vi "ReadVI.vi"(0 "__args":cluster{"targetVi":string}) -> (1 "__return":string, 2 "__errStatus":bool, 3 "__errCode":i32, 4 "__errSource":string)   [LabVIEW 2014]
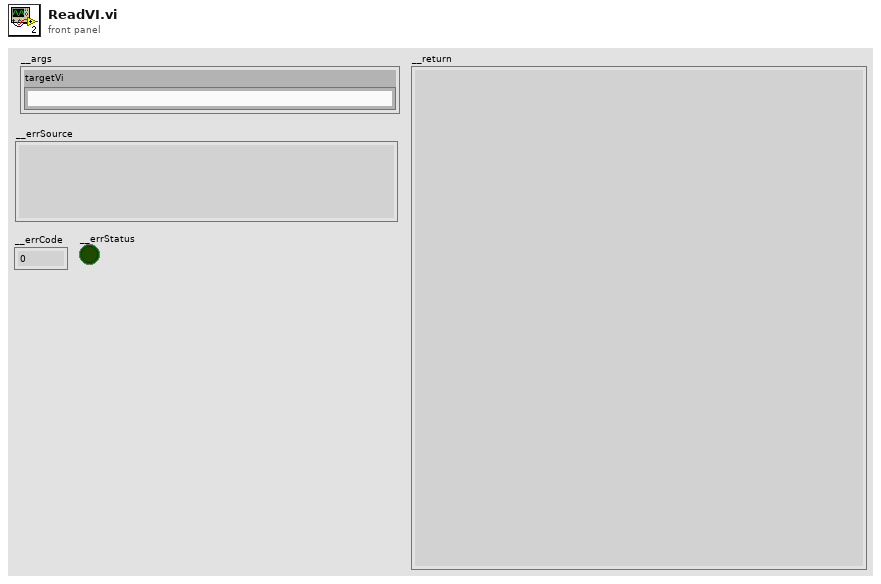
[diagram p1: front panel]
types:
  T1 = typedef "LVBoundsTypeDef.ctl" = cluster{"Width":u32, "Height":u32}
  T2 = typedef "LVPositionTypeDef.ctl" = cluster{"Left":i32, "Top":i32}
  T3 = typedef "LVRectTypeDef.ctl" = cluster{"Left":i16, "Top":i16, "Right":i16, "Bottom":i16}
  T4 = typedef "LVBreakpointStatusEnum.ctl" = enum8{"Cleared Break", "Enabled Break", "Disabled Break"}
  T5 = typedef "LVDataSocketStatusTypeDef.ctl" = cluster{"Code":enum32{"Invalid Status", "Unconnected", "Active", "Idle", "Error", "Connecting"}, "Text":string}
  T6 = typedef "LVKeyNavTypeDef.ctl" = cluster{"Control":bool, "Shift":bool, "Key":string}
  T7 = typedef "LVNumericRepresentation.ctl" = enum32{"Extended Precision", "Double Precision", "Single Precision", "Long", "Word", "Byte", "Unsigned Long", "Unsigned Word", "Unsigned Byte", "Complex Extended", "Complex Double", "Complex Single", "Quad", "Unsigned Quad", "Fixed-Point"}
  T8 = typedef "LVStringsAndValuesArrayTypeDef.ctl" = cluster{"String":string, "Value":ext}[]
  T9 = typedef "LVParallelSchedulesEnum.ctl" = enum8{"Dynamic decreasing", "Dynamic fixed size", "Static block", "Static block-cyclic"}
  T10 = typedef "LVMinMaxIncTypeDef.ctl" = cluster{"Minimum":dbl, "Maximum":dbl, "Increment":dbl}
  T11 = typedef "LVKeyTypeDef.ctl" = cluster{"Focus":bool, "Control":bool, "Shift":bool, "Key":string}
  T12 = typedef "LVOutOfRangeActionTypeDef.ctl" = cluster{"Out of Range Action Minimum":u8, "Out of Range Action Maximum":u8, "Out of Range Action Increment":u8}
  T13 = cluster{"Wire":cluster{"ClassID":u32, "ClassName":string, "IsOnBD?":bool, "Owner":cluster{bool, "UID":i32}, "OwningVI":refnum<vi>, "Bounds":T1, "Height":u32, "Width":u32, "Position":T2, "Left":i32, "Top":i32, "Selected":bool, "Bounds Rect":T3, "UID":i32, "BreakPtStatus":T4, "Desc":string, "Broken?":bool, "Joints[]":cluster{"Position":cluster{"h":i16, "v":i16}, "Flags":i32, "Type":enum32{"LooseEnd", "Endpoint", "Bend", "Junction"}, "Up Joint Index":i16, "Down Joint Index":i16, "Left Joint Index":i16, "Right Joint Index":i16}[], "Label":string, "Probe":refnum<vi>, "Terms[]":i32[], "Width":u32}[], cluster{"ClassID":u32, "ClassName":string, "IsOnBD?":bool, "Owner":cluster{bool, "UID":i32}, "OwningVI":refnum<vi>, "Bounds":T1, "Height":u32, "Width":u32, "Position":T2, "Left":i32, "Top":i32, "Selected":bool, "Bounds Rect":T3, "UID":i32, "Caption":string, "Coerce Dot?":bool, "Wire":i32, "Diagram":i32, "IsHidden":bool, "IsSource":bool, "Name":string}[], cluster{"ClassID":u32, "ClassName":string, "IsOnBD?":bool, "Owner":cluster{bool, "UID":i32}, "OwningVI":refnum<vi>, "Bounds":T1, "Height":u32, "Width":u32, "Position":T2, "Left":i32, "Top":i32, "Selected":bool, "Bounds Rect":T3, "UID":i32, "Input?":bool, "Name":string, "Term":i32}[], cluster{"ClassID":u32, "ClassName":string, "IsOnBD?":bool, "Owner":cluster{bool, "UID":i32}, "OwningVI":refnum<vi>, "Bounds":T1, "Height":u32, "Width":u32, "Position":T2, "Left":i32, "Top":i32, "Selected":bool, "Bounds Rect":T3, "UID":i32, "BreakPtStatus":T4, "Desc":string, "Label":string, "Style":string, "Terms[]":i32[], "FormExpr":string, "FormulaParameters[]":i32[]}[], cluster{"ClassID":u32, "ClassName":string, "IsOnBD?":bool, "Owner":cluster{bool, "UID":i32}, "OwningVI":refnum<vi>, "Bounds":T1, "Height":u32, "Width":u32, "Position":T2, "Left":i32, "Top":i32, "Selected":bool, "Bounds Rect":T3, "UID":i32, "BreakPtStatus":T4, "Desc":string, "Label":string, "Style":string, "Terms[]":i32[], "FormExpr":string, "FormulaParameters[]":i32[]}[], cluster{"ClassID":u32, "ClassName":string, "IsOnBD?":bool, "Owner":cluster{bool, "UID":i32}, "OwningVI":refnum<vi>, "Bounds":T1, "Height":u32, "Width":u32, "Position":T2, "Left":i32, "Top":i32, "Selected":bool, "Bounds Rect":T3, "UID":i32, "BreakPtStatus":T4, "Desc":string, "Label":string, "Style":string, "Terms[]":i32[], "TermHeight":i32, "Invert Inputs?[]":bool[], "Invert Output":bool, "Mode":u32}[], cluster{"ClassID":u32, "ClassName":string, "IsOnBD?":bool, "Owner":cluster{bool, "UID":i32}, "OwningVI":refnum<vi>, "Bounds":T1, "Height":u32, "Width":u32, "Position":T2, "Left":i32, "Top":i32, "Selected":bool, "Bounds Rect":T3, "UID":i32, "BreakPtStatus":T4, "Desc":string, "Label":string, "Style":string, "Terms[]":i32[], "TermHeight":i32, "InputCnt":i32, "InputTerms[]":i32[]}[], cluster{"ClassID":u32, "ClassName":string, "IsOnBD?":bool, "Owner":cluster{bool, "UID":i32}, "OwningVI":refnum<vi>, "Bounds":T1, "Height":u32, "Width":u32, "Position":T2, "Left":i32, "Top":i32, "Selected":bool, "Bounds Rect":T3, "UID":i32, "BreakPtStatus":T4, "Desc":string, "Label":string, "Style":string, "Terms[]":i32[], "TermHeight":i32, "OutputCnt":i32, "OutputTerms[]":i32[]}[], cluster{"ClassID":u32, "ClassName":string, "IsOnBD?":bool, "Owner":cluster{bool, "UID":i32}, "OwningVI":refnum<vi>, "Bounds":T1, "Height":u32, "Width":u32, "Position":T2, "Left":i32, "Top":i32, "Selected":bool, "Bounds Rect":T3, "UID":i32, "Auto-Update":bool, "Blinking":bool, "BuiltInMouseWheelSupport":enum16{"None", "On Hover", "On Key Focus", "On Hover or Key Focus"}, "Caption":refnum<vi>, "ControlIndex":i32, "CtrlRefNodes":refnum<vi>[], "FPB.BindingType":enum32{"Unbound", "Bound To PSP URL", "Bound To Variable Shortcut"}, "FPB.LEDVisible":bool, "FPB.Mode":enum32{"No PSP", "Read", "Write", "Write & Read"}, "FPB.URL":string, "FPB.Status":T5, "DtSktEnbld":bool, "DtSktTagVisible":bool, "DtSktMode":enum32{"No DataSocket", "Publish", "Subscribe", "Publish & Subscribe"}, "DtSktStatus":T5, "DtSktURL":string, "DefVal":variant, "Desc":string, "DisabledEnum":enum8{"Enabled", "Disabled", "Disabled and Grayed Out"}, "KeyNav":T6, "GrowInfo":cluster{"Can Grow Horiz":bool, "Can Grow Vert":bool, "Min Horiz":i16, "Min Vert":i16, "Max Horiz":i16, "Max Vert":i16}, "GrowInfoHorizOnly":bool, "GrowInfoVertOnly":bool, "GrowInfoMaxHoriz":i16, "GrowInfoMaxVert":i16, "GrowInfoMinHoriz":i16, "GrowInfoMinVert":i16, "HasCaption":bool, "Indicator":bool, "InvokeNodes":refnum<vi>[], "IsOnConPane":bool, "Typedef?":enum32{"not a typedef", "typedef", "strict typedef", "class private data"}, "Key Focus":bool, "Label":string, "Locals":refnum<vi>[], "OwningPane":refnum<vi>, "PropNodes":refnum<vi>[], "SkipTabbing":bool, "Style":u32, "SyncDisp":bool, "Terminal":i32, "TipStrip":string, "Typedef Path":path, "Typedef VI":refnum<vi>, "Value":variant, "Visible":bool, "Container Bounds":T1, "Height":u32, "Width":u32, "Is XControl?":bool, "Adapt To Source":bool, "Data Range":T10, "Increment":dbl, "Maximum":dbl, "Minimum":dbl, "DecKeyBind":T11, "IncKeyBind":T11, "Rep":T7, "OutOfRngAction":T12, "OutOfRngActInc":u8, "OutOfRngActMax":u8, "OutOfRngActMin":u8, "UnitLabel":refnum<vi>}[], cluster{"ClassID":u32, "ClassName":string, "IsOnBD?":bool, "Owner":cluster{bool, "UID":i32}, "OwningVI":refnum<vi>, "Bounds":T1, "Height":u32, "Width":u32, "Position":T2, "Left":i32, "Top":i32, "Selected":bool, "Bounds Rect":T3, "UID":i32, "Auto-Update":bool, "Blinking":bool, "BuiltInMouseWheelSupport":enum16{"None", "On Hover", "On Key Focus", "On Hover or Key Focus"}, "Caption":refnum<vi>, "ControlIndex":i32, "CtrlRefNodes":refnum<vi>[], "FPB.BindingType":enum32{"Unbound", "Bound To PSP URL", "Bound To Variable Shortcut"}, "FPB.LEDVisible":bool, "FPB.Mode":enum32{"No PSP", "Read", "Write", "Write & Read"}, "FPB.URL":string, "FPB.Status":T5, "DtSktEnbld":bool, "DtSktTagVisible":bool, "DtSktMode":enum32{"No DataSocket", "Publish", "Subscribe", "Publish & Subscribe"}, "DtSktStatus":T5, "DtSktURL":string, "DefVal":variant, "Desc":string, "DisabledEnum":enum8{"Enabled", "Disabled", "Disabled and Grayed Out"}, "KeyNav":T6, "GrowInfo":cluster{"Can Grow Horiz":bool, "Can Grow Vert":bool, "Min Horiz":i16, "Min Vert":i16, "Max Horiz":i16, "Max Vert":i16}, "GrowInfoHorizOnly":bool, "GrowInfoVertOnly":bool, "GrowInfoMaxHoriz":i16, "GrowInfoMaxVert":i16, "GrowInfoMinHoriz":i16, "GrowInfoMinVert":i16, "HasCaption":bool, "Indicator":bool, "InvokeNodes":refnum<vi>[], "IsOnConPane":bool, "Typedef?":enum32{"not a typedef", "typedef", "strict typedef", "class private data"}, "Key Focus":bool, "Label":string, "Locals":refnum<vi>[], "OwningPane":refnum<vi>, "PropNodes":refnum<vi>[], "SkipTabbing":bool, "Style":u32, "SyncDisp":bool, "Terminal":i32, "TipStrip":string, "Typedef Path":path, "Typedef VI":refnum<vi>, "Value":variant, "Visible":bool, "Container Bounds":T1, "Height":u32, "Width":u32, "Is XControl?":bool, "AllObjs[]":refnum<vi>[], "AutoSize":u32, "ClusterSize":T1, "ClustHeight":u32, "ClustWidth":u32, "Color":u32, "Controls[]":i32[], "Decos[]":refnum<vi>[]}[], cluster{"ClassID":u32, "ClassName":string, "IsOnBD?":bool, "Owner":cluster{bool, "UID":i32}, "OwningVI":refnum<vi>, "Bounds":T1, "Height":u32, "Width":u32, "Position":T2, "Left":i32, "Top":i32, "Selected":bool, "Bounds Rect":T3, "UID":i32, "Auto-Update":bool, "Blinking":bool, "BuiltInMouseWheelSupport":enum16{"None", "On Hover", "On Key Focus", "On Hover or Key Focus"}, "Caption":refnum<vi>, "ControlIndex":i32, "CtrlRefNodes":refnum<vi>[], "FPB.BindingType":enum32{"Unbound", "Bound To PSP URL", "Bound To Variable Shortcut"}, "FPB.LEDVisible":bool, "FPB.Mode":enum32{"No PSP", "Read", "Write", "Write & Read"}, "FPB.URL":string, "FPB.Status":T5, "DtSktEnbld":bool, "DtSktTagVisible":bool, "DtSktMode":enum32{"No DataSocket", "Publish", "Subscribe", "Publish & Subscribe"}, "DtSktStatus":T5, "DtSktURL":string, "DefVal":variant, "Desc":string, "DisabledEnum":enum8{"Enabled", "Disabled", "Disabled and Grayed Out"}, "KeyNav":T6, "GrowInfo":cluster{"Can Grow Horiz":bool, "Can Grow Vert":bool, "Min Horiz":i16, "Min Vert":i16, "Max Horiz":i16, "Max Vert":i16}, "GrowInfoHorizOnly":bool, "GrowInfoVertOnly":bool, "GrowInfoMaxHoriz":i16, "GrowInfoMaxVert":i16, "GrowInfoMinHoriz":i16, "GrowInfoMinVert":i16, "HasCaption":bool, "Indicator":bool, "InvokeNodes":refnum<vi>[], "IsOnConPane":bool, "Typedef?":enum32{"not a typedef", "typedef", "strict typedef", "class private data"}, "Key Focus":bool, "Label":string, "Locals":refnum<vi>[], "OwningPane":refnum<vi>, "PropNodes":refnum<vi>[], "SkipTabbing":bool, "Style":u32, "SyncDisp":bool, "Terminal":i32, "TipStrip":string, "Typedef Path":path, "Typedef VI":refnum<vi>, "Value":variant, "Visible":bool, "Container Bounds":T1, "Height":u32, "Width":u32, "Is XControl?":bool, "Array Element":refnum<vi>, "HorizScroll":bool, "Index Values":u32[], "Index Visible":bool, "Number of Columns":u32, "NumDims":u32, "Number of Rows":u32, "Selection Size []":u32[], "Selection Start []":u32[], "VertScroll":bool}[], cluster{"ClassID":u32, "ClassName":string, "IsOnBD?":bool, "Owner":cluster{bool, "UID":i32}, "OwningVI":refnum<vi>, "Bounds":T1, "Height":u32, "Width":u32, "Position":T2, "Left":i32, "Top":i32, "Selected":bool, "Bounds Rect":T3, "UID":i32, "Auto-Update":bool, "Desc":string, "Typedef?":enum32{"not a typedef", "typedef", "strict typedef", "class private data"}, "Label":string, "Terminal":i32, "TipStrip":string, "Typedef Path":path, "Typedef VI":refnum<vi>, "Value":variant, "Adapt To Entered Data":bool, "Representation":T7, "DigDisp":refnum<vi>, "Items[]":string[], "Allow Undefined Values?":bool, "Strings And Values[]":T8}[], cluster{"ClassID":u32, "ClassName":string, "IsOnBD?":bool, "Owner":cluster{bool, "UID":i32}, "OwningVI":refnum<vi>, "Bounds":T1, "Height":u32, "Width":u32, "Position":T2, "Left":i32, "Top":i32, "Selected":bool, "Bounds Rect":T3, "UID":i32, "BreakPtStatus":T4, "Desc":string, "Label":string, "Style":string, "Terms[]":i32[], "BadSubVILinkage":bool, "GrowTerms":string[], "SkipSbrtCall":bool, "CloseFPAfterCall":bool, "Open FP On Load":bool, "Show FP On Call":bool, "SuspendOnCall":bool, "TermVis":bool, "VIName":string, "VIPath":path, "VI Ref":refnum<vi>, "ViewAsIcon":bool}[], cluster{"ClassID":u32, "ClassName":string, "IsOnBD?":bool, "Owner":cluster{bool, "UID":i32}, "OwningVI":refnum<vi>, "Bounds":T1, "Height":u32, "Width":u32, "Position":T2, "Left":i32, "Top":i32, "Selected":bool, "Bounds Rect":T3, "UID":i32, "InsideTerms[]":i32[], "Outer Term":i32, "RightReg":i32}[], cluster{"ClassID":u32, "ClassName":string, "IsOnBD?":bool, "Owner":cluster{bool, "UID":i32}, "OwningVI":refnum<vi>, "Bounds":T1, "Height":u32, "Width":u32, "Position":T2, "Left":i32, "Top":i32, "Selected":bool, "Bounds Rect":T3, "UID":i32, "InsideTerms[]":i32[], "Outer Term":i32, "LeftRegs[]":i32[]}[], cluster{"ClassID":u32, "ClassName":string, "IsOnBD?":bool, "Owner":cluster{bool, "UID":i32}, "OwningVI":refnum<vi>, "Bounds":T1, "Height":u32, "Width":u32, "Position":T2, "Left":i32, "Top":i32, "Selected":bool, "Bounds Rect":T3, "UID":i32, "BreakPtStatus":T4, "Desc":string, "Label":string, "Style":string, "Terms[]":i32[], "AutoSize":bool, "Content Rect":T3, "Diagrams":refnum<vi>[], "Fix Contents":bool, "Frame Size":T1, "AutoSharedCloneAllocStrategyEnabled":bool, "PreAllocSharedClones":bool, "SubDiagLbl Vis":bool, "Tunnels[]":i32[], "Diagram":i32, "LpCounter":refnum<vi>, "ShiftRegs[]":i32[], "LpEndRef":refnum<vi>, "StopIfTrue":bool}[], cluster{"ClassID":u32, "ClassName":string, "IsOnBD?":bool, "Owner":cluster{bool, "UID":i32}, "OwningVI":refnum<vi>, "Bounds":T1, "Height":u32, "Width":u32, "Position":T2, "Left":i32, "Top":i32, "Selected":bool, "Bounds Rect":T3, "UID":i32, "BreakPtStatus":T4, "Desc":string, "Label":string, "Style":string, "Terms[]":i32[], "AutoSize":bool, "Content Rect":T3, "Diagrams":refnum<vi>[], "Fix Contents":bool, "Frame Size":T1, "AutoSharedCloneAllocStrategyEnabled":bool, "PreAllocSharedClones":bool, "SubDiagLbl Vis":bool, "Tunnels[]":i32[], "Diagram":i32, "LpCounter":refnum<vi>, "ShiftRegs[]":i32[], "ChunkSizeTunnel":refnum<vi>, "PTunnel":refnum<vi>, "HasConditionalTerm":bool, "DebuggingAllowed":bool, "IsParallelismEnabled":bool, "LpCount":refnum<vi>, "LpEndRef":refnum<vi>, "NumStaticParWorkers":i32, "ParallelSchedule":T9, "StopIfTrue":bool}[], cluster{"ClassID":u32, "ClassName":string, "IsOnBD?":bool, "Owner":cluster{bool, "UID":i32}, "OwningVI":refnum<vi>, "Bounds":T1, "Height":u32, "Width":u32, "Position":T2, "Left":i32, "Top":i32, "Selected":bool, "Bounds Rect":T3, "UID":i32, "AllObjs[]":refnum<vi>[], "BreakPtStatus":T4, "Color":u32, "Decos[]":refnum<vi>[], "FiringOrder":refnum<vi>[], "Nodes[]":refnum<vi>[], "SubDiag Label":refnum<vi>, "SubVIs[]":refnum<vi>[], "Wires[]":refnum<vi>[], "VisBounds":T1}[], cluster{"ClassID":u32, "ClassName":string, "IsOnBD?":bool, "Owner":cluster{bool, "UID":i32}, "OwningVI":refnum<vi>, "Bounds":T1, "Height":u32, "Width":u32, "Position":T2, "Left":i32, "Top":i32, "Selected":bool, "Bounds Rect":T3, "UID":i32, "AllObjs[]":refnum<vi>[], "Controls[]":i32[], "Decos[]":refnum<vi>[], "DeferPanUpdts":bool, "Panes[]":refnum<vi>[], "SelList[]":refnum<vi>[], "Splitters[]":refnum<vi>[]}[], cluster{"ClassID":u32, "ClassName":string, "IsOnBD?":bool, "Owner":cluster{bool, "UID":i32}, "OwningVI":refnum<vi>, "Bounds":T1, "Height":u32, "Width":u32, "Position":T2, "Left":i32, "Top":i32, "Selected":bool, "Bounds Rect":T3, "UID":i32, "InsideTerms[]":i32[], "Outer Term":i32}[]}
  T14 = cluster{"ClassID":u32, "ClassName":string, "IsOnBD?":bool, "Owner":cluster{bool, "UID":i32}, "OwningVI":refnum<vi>, "Bounds":T1, "Height":u32, "Width":u32, "Position":T2, "Left":i32, "Top":i32, "Selected":bool, "Bounds Rect":T3, "UID":i32, "BreakPtStatus":T4, "Desc":string, "Broken?":bool, "Joints[]":cluster{"Position":cluster{"h":i16, "v":i16}, "Flags":i32, "Type":enum32{"LooseEnd", "Endpoint", "Bend", "Junction"}, "Up Joint Index":i16, "Down Joint Index":i16, "Left Joint Index":i16, "Right Joint Index":i16}[], "Label":string, "Probe":refnum<vi>, "Terms[]":i32[], "Width":u32}[]
  T15 = cluster{"ClassID":u32, "ClassName":string, "IsOnBD?":bool, "Owner":cluster{bool, "UID":i32}, "OwningVI":refnum<vi>, "Bounds":T1, "Height":u32, "Width":u32, "Position":T2, "Left":i32, "Top":i32, "Selected":bool, "Bounds Rect":T3, "UID":i32, "Caption":string, "Coerce Dot?":bool, "Wire":i32, "Diagram":i32, "IsHidden":bool, "IsSource":bool, "Name":string}[]
  T16 = cluster{"ClassID":u32, "ClassName":string, "IsOnBD?":bool, "Owner":cluster{bool, "UID":i32}, "OwningVI":refnum<vi>, "Bounds":T1, "Height":u32, "Width":u32, "Position":T2, "Left":i32, "Top":i32, "Selected":bool, "Bounds Rect":T3, "UID":i32, "Input?":bool, "Name":string, "Term":i32}[]
  T17 = cluster{"ClassID":u32, "ClassName":string, "IsOnBD?":bool, "Owner":cluster{bool, "UID":i32}, "OwningVI":refnum<vi>, "Bounds":T1, "Height":u32, "Width":u32, "Position":T2, "Left":i32, "Top":i32, "Selected":bool, "Bounds Rect":T3, "UID":i32, "BreakPtStatus":T4, "Desc":string, "Label":string, "Style":string, "Terms[]":i32[], "FormExpr":string, "FormulaParameters[]":i32[]}[]
  T18 = cluster{"ClassID":u32, "ClassName":string, "IsOnBD?":bool, "Owner":cluster{bool, "UID":i32}, "OwningVI":refnum<vi>, "Bounds":T1, "Height":u32, "Width":u32, "Position":T2, "Left":i32, "Top":i32, "Selected":bool, "Bounds Rect":T3, "UID":i32, "BreakPtStatus":T4, "Desc":string, "Label":string, "Style":string, "Terms[]":i32[], "TermHeight":i32, "Invert Inputs?[]":bool[], "Invert Output":bool, "Mode":u32}[]
  T19 = cluster{"ClassID":u32, "ClassName":string, "IsOnBD?":bool, "Owner":cluster{bool, "UID":i32}, "OwningVI":refnum<vi>, "Bounds":T1, "Height":u32, "Width":u32, "Position":T2, "Left":i32, "Top":i32, "Selected":bool, "Bounds Rect":T3, "UID":i32, "BreakPtStatus":T4, "Desc":string, "Label":string, "Style":string, "Terms[]":i32[], "TermHeight":i32, "InputCnt":i32, "InputTerms[]":i32[]}[]
  T20 = cluster{"ClassID":u32, "ClassName":string, "IsOnBD?":bool, "Owner":cluster{bool, "UID":i32}, "OwningVI":refnum<vi>, "Bounds":T1, "Height":u32, "Width":u32, "Position":T2, "Left":i32, "Top":i32, "Selected":bool, "Bounds Rect":T3, "UID":i32, "BreakPtStatus":T4, "Desc":string, "Label":string, "Style":string, "Terms[]":i32[], "TermHeight":i32, "OutputCnt":i32, "OutputTerms[]":i32[]}[]
  T21 = cluster{"ClassID":u32, "ClassName":string, "IsOnBD?":bool, "Owner":cluster{bool, "UID":i32}, "OwningVI":refnum<vi>, "Bounds":T1, "Height":u32, "Width":u32, "Position":T2, "Left":i32, "Top":i32, "Selected":bool, "Bounds Rect":T3, "UID":i32, "Auto-Update":bool, "Blinking":bool, "BuiltInMouseWheelSupport":enum16{"None", "On Hover", "On Key Focus", "On Hover or Key Focus"}, "Caption":refnum<vi>, "ControlIndex":i32, "CtrlRefNodes":refnum<vi>[], "FPB.BindingType":enum32{"Unbound", "Bound To PSP URL", "Bound To Variable Shortcut"}, "FPB.LEDVisible":bool, "FPB.Mode":enum32{"No PSP", "Read", "Write", "Write & Read"}, "FPB.URL":string, "FPB.Status":T5, "DtSktEnbld":bool, "DtSktTagVisible":bool, "DtSktMode":enum32{"No DataSocket", "Publish", "Subscribe", "Publish & Subscribe"}, "DtSktStatus":T5, "DtSktURL":string, "DefVal":variant, "Desc":string, "DisabledEnum":enum8{"Enabled", "Disabled", "Disabled and Grayed Out"}, "KeyNav":T6, "GrowInfo":cluster{"Can Grow Horiz":bool, "Can Grow Vert":bool, "Min Horiz":i16, "Min Vert":i16, "Max Horiz":i16, "Max Vert":i16}, "GrowInfoHorizOnly":bool, "GrowInfoVertOnly":bool, "GrowInfoMaxHoriz":i16, "GrowInfoMaxVert":i16, "GrowInfoMinHoriz":i16, "GrowInfoMinVert":i16, "HasCaption":bool, "Indicator":bool, "InvokeNodes":refnum<vi>[], "IsOnConPane":bool, "Typedef?":enum32{"not a typedef", "typedef", "strict typedef", "class private data"}, "Key Focus":bool, "Label":string, "Locals":refnum<vi>[], "OwningPane":refnum<vi>, "PropNodes":refnum<vi>[], "SkipTabbing":bool, "Style":u32, "SyncDisp":bool, "Terminal":i32, "TipStrip":string, "Typedef Path":path, "Typedef VI":refnum<vi>, "Value":variant, "Visible":bool, "Container Bounds":T1, "Height":u32, "Width":u32, "Is XControl?":bool, "Adapt To Source":bool, "Data Range":T10, "Increment":dbl, "Maximum":dbl, "Minimum":dbl, "DecKeyBind":T11, "IncKeyBind":T11, "Rep":T7, "OutOfRngAction":T12, "OutOfRngActInc":u8, "OutOfRngActMax":u8, "OutOfRngActMin":u8, "UnitLabel":refnum<vi>}[]
  T22 = cluster{"ClassID":u32, "ClassName":string, "IsOnBD?":bool, "Owner":cluster{bool, "UID":i32}, "OwningVI":refnum<vi>, "Bounds":T1, "Height":u32, "Width":u32, "Position":T2, "Left":i32, "Top":i32, "Selected":bool, "Bounds Rect":T3, "UID":i32, "Auto-Update":bool, "Blinking":bool, "BuiltInMouseWheelSupport":enum16{"None", "On Hover", "On Key Focus", "On Hover or Key Focus"}, "Caption":refnum<vi>, "ControlIndex":i32, "CtrlRefNodes":refnum<vi>[], "FPB.BindingType":enum32{"Unbound", "Bound To PSP URL", "Bound To Variable Shortcut"}, "FPB.LEDVisible":bool, "FPB.Mode":enum32{"No PSP", "Read", "Write", "Write & Read"}, "FPB.URL":string, "FPB.Status":T5, "DtSktEnbld":bool, "DtSktTagVisible":bool, "DtSktMode":enum32{"No DataSocket", "Publish", "Subscribe", "Publish & Subscribe"}, "DtSktStatus":T5, "DtSktURL":string, "DefVal":variant, "Desc":string, "DisabledEnum":enum8{"Enabled", "Disabled", "Disabled and Grayed Out"}, "KeyNav":T6, "GrowInfo":cluster{"Can Grow Horiz":bool, "Can Grow Vert":bool, "Min Horiz":i16, "Min Vert":i16, "Max Horiz":i16, "Max Vert":i16}, "GrowInfoHorizOnly":bool, "GrowInfoVertOnly":bool, "GrowInfoMaxHoriz":i16, "GrowInfoMaxVert":i16, "GrowInfoMinHoriz":i16, "GrowInfoMinVert":i16, "HasCaption":bool, "Indicator":bool, "InvokeNodes":refnum<vi>[], "IsOnConPane":bool, "Typedef?":enum32{"not a typedef", "typedef", "strict typedef", "class private data"}, "Key Focus":bool, "Label":string, "Locals":refnum<vi>[], "OwningPane":refnum<vi>, "PropNodes":refnum<vi>[], "SkipTabbing":bool, "Style":u32, "SyncDisp":bool, "Terminal":i32, "TipStrip":string, "Typedef Path":path, "Typedef VI":refnum<vi>, "Value":variant, "Visible":bool, "Container Bounds":T1, "Height":u32, "Width":u32, "Is XControl?":bool, "AllObjs[]":refnum<vi>[], "AutoSize":u32, "ClusterSize":T1, "ClustHeight":u32, "ClustWidth":u32, "Color":u32, "Controls[]":i32[], "Decos[]":refnum<vi>[]}[]
  T23 = cluster{"ClassID":u32, "ClassName":string, "IsOnBD?":bool, "Owner":cluster{bool, "UID":i32}, "OwningVI":refnum<vi>, "Bounds":T1, "Height":u32, "Width":u32, "Position":T2, "Left":i32, "Top":i32, "Selected":bool, "Bounds Rect":T3, "UID":i32, "Auto-Update":bool, "Blinking":bool, "BuiltInMouseWheelSupport":enum16{"None", "On Hover", "On Key Focus", "On Hover or Key Focus"}, "Caption":refnum<vi>, "ControlIndex":i32, "CtrlRefNodes":refnum<vi>[], "FPB.BindingType":enum32{"Unbound", "Bound To PSP URL", "Bound To Variable Shortcut"}, "FPB.LEDVisible":bool, "FPB.Mode":enum32{"No PSP", "Read", "Write", "Write & Read"}, "FPB.URL":string, "FPB.Status":T5, "DtSktEnbld":bool, "DtSktTagVisible":bool, "DtSktMode":enum32{"No DataSocket", "Publish", "Subscribe", "Publish & Subscribe"}, "DtSktStatus":T5, "DtSktURL":string, "DefVal":variant, "Desc":string, "DisabledEnum":enum8{"Enabled", "Disabled", "Disabled and Grayed Out"}, "KeyNav":T6, "GrowInfo":cluster{"Can Grow Horiz":bool, "Can Grow Vert":bool, "Min Horiz":i16, "Min Vert":i16, "Max Horiz":i16, "Max Vert":i16}, "GrowInfoHorizOnly":bool, "GrowInfoVertOnly":bool, "GrowInfoMaxHoriz":i16, "GrowInfoMaxVert":i16, "GrowInfoMinHoriz":i16, "GrowInfoMinVert":i16, "HasCaption":bool, "Indicator":bool, "InvokeNodes":refnum<vi>[], "IsOnConPane":bool, "Typedef?":enum32{"not a typedef", "typedef", "strict typedef", "class private data"}, "Key Focus":bool, "Label":string, "Locals":refnum<vi>[], "OwningPane":refnum<vi>, "PropNodes":refnum<vi>[], "SkipTabbing":bool, "Style":u32, "SyncDisp":bool, "Terminal":i32, "TipStrip":string, "Typedef Path":path, "Typedef VI":refnum<vi>, "Value":variant, "Visible":bool, "Container Bounds":T1, "Height":u32, "Width":u32, "Is XControl?":bool, "Array Element":refnum<vi>, "HorizScroll":bool, "Index Values":u32[], "Index Visible":bool, "Number of Columns":u32, "NumDims":u32, "Number of Rows":u32, "Selection Size []":u32[], "Selection Start []":u32[], "VertScroll":bool}[]
  T24 = cluster{"ClassID":u32, "ClassName":string, "IsOnBD?":bool, "Owner":cluster{bool, "UID":i32}, "OwningVI":refnum<vi>, "Bounds":T1, "Height":u32, "Width":u32, "Position":T2, "Left":i32, "Top":i32, "Selected":bool, "Bounds Rect":T3, "UID":i32, "Auto-Update":bool, "Desc":string, "Typedef?":enum32{"not a typedef", "typedef", "strict typedef", "class private data"}, "Label":string, "Terminal":i32, "TipStrip":string, "Typedef Path":path, "Typedef VI":refnum<vi>, "Value":variant, "Adapt To Entered Data":bool, "Representation":T7, "DigDisp":refnum<vi>, "Items[]":string[], "Allow Undefined Values?":bool, "Strings And Values[]":T8}[]
  T25 = cluster{"ClassID":u32, "ClassName":string, "IsOnBD?":bool, "Owner":cluster{bool, "UID":i32}, "OwningVI":refnum<vi>, "Bounds":T1, "Height":u32, "Width":u32, "Position":T2, "Left":i32, "Top":i32, "Selected":bool, "Bounds Rect":T3, "UID":i32, "BreakPtStatus":T4, "Desc":string, "Label":string, "Style":string, "Terms[]":i32[], "BadSubVILinkage":bool, "GrowTerms":string[], "SkipSbrtCall":bool, "CloseFPAfterCall":bool, "Open FP On Load":bool, "Show FP On Call":bool, "SuspendOnCall":bool, "TermVis":bool, "VIName":string, "VIPath":path, "VI Ref":refnum<vi>, "ViewAsIcon":bool}[]
  T26 = cluster{"ClassID":u32, "ClassName":string, "IsOnBD?":bool, "Owner":cluster{bool, "UID":i32}, "OwningVI":refnum<vi>, "Bounds":T1, "Height":u32, "Width":u32, "Position":T2, "Left":i32, "Top":i32, "Selected":bool, "Bounds Rect":T3, "UID":i32, "InsideTerms[]":i32[], "Outer Term":i32, "RightReg":i32}[]
  T27 = cluster{"ClassID":u32, "ClassName":string, "IsOnBD?":bool, "Owner":cluster{bool, "UID":i32}, "OwningVI":refnum<vi>, "Bounds":T1, "Height":u32, "Width":u32, "Position":T2, "Left":i32, "Top":i32, "Selected":bool, "Bounds Rect":T3, "UID":i32, "InsideTerms[]":i32[], "Outer Term":i32, "LeftRegs[]":i32[]}[]
  T28 = cluster{"ClassID":u32, "ClassName":string, "IsOnBD?":bool, "Owner":cluster{bool, "UID":i32}, "OwningVI":refnum<vi>, "Bounds":T1, "Height":u32, "Width":u32, "Position":T2, "Left":i32, "Top":i32, "Selected":bool, "Bounds Rect":T3, "UID":i32, "BreakPtStatus":T4, "Desc":string, "Label":string, "Style":string, "Terms[]":i32[], "AutoSize":bool, "Content Rect":T3, "Diagrams":refnum<vi>[], "Fix Contents":bool, "Frame Size":T1, "AutoSharedCloneAllocStrategyEnabled":bool, "PreAllocSharedClones":bool, "SubDiagLbl Vis":bool, "Tunnels[]":i32[], "Diagram":i32, "LpCounter":refnum<vi>, "ShiftRegs[]":i32[], "LpEndRef":refnum<vi>, "StopIfTrue":bool}[]
  T29 = cluster{"ClassID":u32, "ClassName":string, "IsOnBD?":bool, "Owner":cluster{bool, "UID":i32}, "OwningVI":refnum<vi>, "Bounds":T1, "Height":u32, "Width":u32, "Position":T2, "Left":i32, "Top":i32, "Selected":bool, "Bounds Rect":T3, "UID":i32, "BreakPtStatus":T4, "Desc":string, "Label":string, "Style":string, "Terms[]":i32[], "AutoSize":bool, "Content Rect":T3, "Diagrams":refnum<vi>[], "Fix Contents":bool, "Frame Size":T1, "AutoSharedCloneAllocStrategyEnabled":bool, "PreAllocSharedClones":bool, "SubDiagLbl Vis":bool, "Tunnels[]":i32[], "Diagram":i32, "LpCounter":refnum<vi>, "ShiftRegs[]":i32[], "ChunkSizeTunnel":refnum<vi>, "PTunnel":refnum<vi>, "HasConditionalTerm":bool, "DebuggingAllowed":bool, "IsParallelismEnabled":bool, "LpCount":refnum<vi>, "LpEndRef":refnum<vi>, "NumStaticParWorkers":i32, "ParallelSchedule":T9, "StopIfTrue":bool}[]
  T30 = cluster{"ClassID":u32, "ClassName":string, "IsOnBD?":bool, "Owner":cluster{bool, "UID":i32}, "OwningVI":refnum<vi>, "Bounds":T1, "Height":u32, "Width":u32, "Position":T2, "Left":i32, "Top":i32, "Selected":bool, "Bounds Rect":T3, "UID":i32, "AllObjs[]":refnum<vi>[], "BreakPtStatus":T4, "Color":u32, "Decos[]":refnum<vi>[], "FiringOrder":refnum<vi>[], "Nodes[]":refnum<vi>[], "SubDiag Label":refnum<vi>, "SubVIs[]":refnum<vi>[], "Wires[]":refnum<vi>[], "VisBounds":T1}[]
  T31 = cluster{"ClassID":u32, "ClassName":string, "IsOnBD?":bool, "Owner":cluster{bool, "UID":i32}, "OwningVI":refnum<vi>, "Bounds":T1, "Height":u32, "Width":u32, "Position":T2, "Left":i32, "Top":i32, "Selected":bool, "Bounds Rect":T3, "UID":i32, "AllObjs[]":refnum<vi>[], "Controls[]":i32[], "Decos[]":refnum<vi>[], "DeferPanUpdts":bool, "Panes[]":refnum<vi>[], "SelList[]":refnum<vi>[], "Splitters[]":refnum<vi>[]}[]
  T32 = cluster{"ClassID":u32, "ClassName":string, "IsOnBD?":bool, "Owner":cluster{bool, "UID":i32}, "OwningVI":refnum<vi>, "Bounds":T1, "Height":u32, "Width":u32, "Position":T2, "Left":i32, "Top":i32, "Selected":bool, "Bounds Rect":T3, "UID":i32, "InsideTerms[]":i32[], "Outer Term":i32}[]
  T33 = cluster{cluster{"Controls[]":i32[]}[], "Wire":cluster{"ClassID":u32, "ClassName":string, "IsOnBD?":bool, "Owner":cluster{bool, "UID":i32}, "OwningVI":refnum<vi>, "Bounds":T1, "Height":u32, "Width":u32, "Position":T2, "Left":i32, "Top":i32, "Selected":bool, "Bounds Rect":T3, "UID":i32, "BreakPtStatus":T4, "Desc":string, "Broken?":bool, "Joints[]":cluster{"Position":cluster{"h":i16, "v":i16}, "Flags":i32, "Type":enum32{"LooseEnd", "Endpoint", "Bend", "Junction"}, "Up Joint Index":i16, "Down Joint Index":i16, "Left Joint Index":i16, "Right Joint Index":i16}[], "Label":string, "Probe":refnum<vi>, "Terms[]":i32[], "Width":u32}[], cluster{"ClassID":u32, "ClassName":string, "IsOnBD?":bool, "Owner":cluster{bool, "UID":i32}, "OwningVI":refnum<vi>, "Bounds":T1, "Height":u32, "Width":u32, "Position":T2, "Left":i32, "Top":i32, "Selected":bool, "Bounds Rect":T3, "UID":i32, "Caption":string, "Coerce Dot?":bool, "Wire":i32, "Diagram":i32, "IsHidden":bool, "IsSource":bool, "Name":string}[], cluster{"ClassID":u32, "ClassName":string, "IsOnBD?":bool, "Owner":cluster{bool, "UID":i32}, "OwningVI":refnum<vi>, "Bounds":T1, "Height":u32, "Width":u32, "Position":T2, "Left":i32, "Top":i32, "Selected":bool, "Bounds Rect":T3, "UID":i32, "Input?":bool, "Name":string, "Term":i32}[], cluster{"ClassID":u32, "ClassName":string, "IsOnBD?":bool, "Owner":cluster{bool, "UID":i32}, "OwningVI":refnum<vi>, "Bounds":T1, "Height":u32, "Width":u32, "Position":T2, "Left":i32, "Top":i32, "Selected":bool, "Bounds Rect":T3, "UID":i32, "BreakPtStatus":T4, "Desc":string, "Label":string, "Style":string, "Terms[]":i32[], "FormExpr":string, "FormulaParameters[]":i32[]}[], cluster{"ClassID":u32, "ClassName":string, "IsOnBD?":bool, "Owner":cluster{bool, "UID":i32}, "OwningVI":refnum<vi>, "Bounds":T1, "Height":u32, "Width":u32, "Position":T2, "Left":i32, "Top":i32, "Selected":bool, "Bounds Rect":T3, "UID":i32, "BreakPtStatus":T4, "Desc":string, "Label":string, "Style":string, "Terms[]":i32[], "FormExpr":string, "FormulaParameters[]":i32[]}[], cluster{"ClassID":u32, "ClassName":string, "IsOnBD?":bool, "Owner":cluster{bool, "UID":i32}, "OwningVI":refnum<vi>, "Bounds":T1, "Height":u32, "Width":u32, "Position":T2, "Left":i32, "Top":i32, "Selected":bool, "Bounds Rect":T3, "UID":i32, "BreakPtStatus":T4, "Desc":string, "Label":string, "Style":string, "Terms[]":i32[], "TermHeight":i32, "Invert Inputs?[]":bool[], "Invert Output":bool, "Mode":u32}[], cluster{"ClassID":u32, "ClassName":string, "IsOnBD?":bool, "Owner":cluster{bool, "UID":i32}, "OwningVI":refnum<vi>, "Bounds":T1, "Height":u32, "Width":u32, "Position":T2, "Left":i32, "Top":i32, "Selected":bool, "Bounds Rect":T3, "UID":i32, "BreakPtStatus":T4, "Desc":string, "Label":string, "Style":string, "Terms[]":i32[], "TermHeight":i32, "InputCnt":i32, "InputTerms[]":i32[]}[], cluster{"ClassID":u32, "ClassName":string, "IsOnBD?":bool, "Owner":cluster{bool, "UID":i32}, "OwningVI":refnum<vi>, "Bounds":T1, "Height":u32, "Width":u32, "Position":T2, "Left":i32, "Top":i32, "Selected":bool, "Bounds Rect":T3, "UID":i32, "BreakPtStatus":T4, "Desc":string, "Label":string, "Style":string, "Terms[]":i32[], "TermHeight":i32, "OutputCnt":i32, "OutputTerms[]":i32[]}[], cluster{"ClassID":u32, "ClassName":string, "IsOnBD?":bool, "Owner":cluster{bool, "UID":i32}, "OwningVI":refnum<vi>, "Bounds":T1, "Height":u32, "Width":u32, "Position":T2, "Left":i32, "Top":i32, "Selected":bool, "Bounds Rect":T3, "UID":i32, "Auto-Update":bool, "Blinking":bool, "BuiltInMouseWheelSupport":enum16{"None", "On Hover", "On Key Focus", "On Hover or Key Focus"}, "Caption":refnum<vi>, "ControlIndex":i32, "CtrlRefNodes":refnum<vi>[], "FPB.BindingType":enum32{"Unbound", "Bound To PSP URL", "Bound To Variable Shortcut"}, "FPB.LEDVisible":bool, "FPB.Mode":enum32{"No PSP", "Read", "Write", "Write & Read"}, "FPB.URL":string, "FPB.Status":T5, "DtSktEnbld":bool, "DtSktTagVisible":bool, "DtSktMode":enum32{"No DataSocket", "Publish", "Subscribe", "Publish & Subscribe"}, "DtSktStatus":T5, "DtSktURL":string, "DefVal":variant, "Desc":string, "DisabledEnum":enum8{"Enabled", "Disabled", "Disabled and Grayed Out"}, "KeyNav":T6, "GrowInfo":cluster{"Can Grow Horiz":bool, "Can Grow Vert":bool, "Min Horiz":i16, "Min Vert":i16, "Max Horiz":i16, "Max Vert":i16}, "GrowInfoHorizOnly":bool, "GrowInfoVertOnly":bool, "GrowInfoMaxHoriz":i16, "GrowInfoMaxVert":i16, "GrowInfoMinHoriz":i16, "GrowInfoMinVert":i16, "HasCaption":bool, "Indicator":bool, "InvokeNodes":refnum<vi>[], "IsOnConPane":bool, "Typedef?":enum32{"not a typedef", "typedef", "strict typedef", "class private data"}, "Key Focus":bool, "Label":string, "Locals":refnum<vi>[], "OwningPane":refnum<vi>, "PropNodes":refnum<vi>[], "SkipTabbing":bool, "Style":u32, "SyncDisp":bool, "Terminal":i32, "TipStrip":string, "Typedef Path":path, "Typedef VI":refnum<vi>, "Value":variant, "Visible":bool, "Container Bounds":T1, "Height":u32, "Width":u32, "Is XControl?":bool, "Adapt To Source":bool, "Data Range":T10, "Increment":dbl, "Maximum":dbl, "Minimum":dbl, "DecKeyBind":T11, "IncKeyBind":T11, "Rep":T7, "OutOfRngAction":T12, "OutOfRngActInc":u8, "OutOfRngActMax":u8, "OutOfRngActMin":u8, "UnitLabel":refnum<vi>}[], cluster{"ClassID":u32, "ClassName":string, "IsOnBD?":bool, "Owner":cluster{bool, "UID":i32}, "OwningVI":refnum<vi>, "Bounds":T1, "Height":u32, "Width":u32, "Position":T2, "Left":i32, "Top":i32, "Selected":bool, "Bounds Rect":T3, "UID":i32, "Auto-Update":bool, "Blinking":bool, "BuiltInMouseWheelSupport":enum16{"None", "On Hover", "On Key Focus", "On Hover or Key Focus"}, "Caption":refnum<vi>, "ControlIndex":i32, "CtrlRefNodes":refnum<vi>[], "FPB.BindingType":enum32{"Unbound", "Bound To PSP URL", "Bound To Variable Shortcut"}, "FPB.LEDVisible":bool, "FPB.Mode":enum32{"No PSP", "Read", "Write", "Write & Read"}, "FPB.URL":string, "FPB.Status":T5, "DtSktEnbld":bool, "DtSktTagVisible":bool, "DtSktMode":enum32{"No DataSocket", "Publish", "Subscribe", "Publish & Subscribe"}, "DtSktStatus":T5, "DtSktURL":string, "DefVal":variant, "Desc":string, "DisabledEnum":enum8{"Enabled", "Disabled", "Disabled and Grayed Out"}, "KeyNav":T6, "GrowInfo":cluster{"Can Grow Horiz":bool, "Can Grow Vert":bool, "Min Horiz":i16, "Min Vert":i16, "Max Horiz":i16, "Max Vert":i16}, "GrowInfoHorizOnly":bool, "GrowInfoVertOnly":bool, "GrowInfoMaxHoriz":i16, "GrowInfoMaxVert":i16, "GrowInfoMinHoriz":i16, "GrowInfoMinVert":i16, "HasCaption":bool, "Indicator":bool, "InvokeNodes":refnum<vi>[], "IsOnConPane":bool, "Typedef?":enum32{"not a typedef", "typedef", "strict typedef", "class private data"}, "Key Focus":bool, "Label":string, "Locals":refnum<vi>[], "OwningPane":refnum<vi>, "PropNodes":refnum<vi>[], "SkipTabbing":bool, "Style":u32, "SyncDisp":bool, "Terminal":i32, "TipStrip":string, "Typedef Path":path, "Typedef VI":refnum<vi>, "Value":variant, "Visible":bool, "Container Bounds":T1, "Height":u32, "Width":u32, "Is XControl?":bool, "AllObjs[]":refnum<vi>[], "AutoSize":u32, "ClusterSize":T1, "ClustHeight":u32, "ClustWidth":u32, "Color":u32, "Controls[]":i32[], "Decos[]":refnum<vi>[]}[], cluster{"ClassID":u32, "ClassName":string, "IsOnBD?":bool, "Owner":cluster{bool, "UID":i32}, "OwningVI":refnum<vi>, "Bounds":T1, "Height":u32, "Width":u32, "Position":T2, "Left":i32, "Top":i32, "Selected":bool, "Bounds Rect":T3, "UID":i32, "Auto-Update":bool, "Blinking":bool, "BuiltInMouseWheelSupport":enum16{"None", "On Hover", "On Key Focus", "On Hover or Key Focus"}, "Caption":refnum<vi>, "ControlIndex":i32, "CtrlRefNodes":refnum<vi>[], "FPB.BindingType":enum32{"Unbound", "Bound To PSP URL", "Bound To Variable Shortcut"}, "FPB.LEDVisible":bool, "FPB.Mode":enum32{"No PSP", "Read", "Write", "Write & Read"}, "FPB.URL":string, "FPB.Status":T5, "DtSktEnbld":bool, "DtSktTagVisible":bool, "DtSktMode":enum32{"No DataSocket", "Publish", "Subscribe", "Publish & Subscribe"}, "DtSktStatus":T5, "DtSktURL":string, "DefVal":variant, "Desc":string, "DisabledEnum":enum8{"Enabled", "Disabled", "Disabled and Grayed Out"}, "KeyNav":T6, "GrowInfo":cluster{"Can Grow Horiz":bool, "Can Grow Vert":bool, "Min Horiz":i16, "Min Vert":i16, "Max Horiz":i16, "Max Vert":i16}, "GrowInfoHorizOnly":bool, "GrowInfoVertOnly":bool, "GrowInfoMaxHoriz":i16, "GrowInfoMaxVert":i16, "GrowInfoMinHoriz":i16, "GrowInfoMinVert":i16, "HasCaption":bool, "Indicator":bool, "InvokeNodes":refnum<vi>[], "IsOnConPane":bool, "Typedef?":enum32{"not a typedef", "typedef", "strict typedef", "class private data"}, "Key Focus":bool, "Label":string, "Locals":refnum<vi>[], "OwningPane":refnum<vi>, "PropNodes":refnum<vi>[], "SkipTabbing":bool, "Style":u32, "SyncDisp":bool, "Terminal":i32, "TipStrip":string, "Typedef Path":path, "Typedef VI":refnum<vi>, "Value":variant, "Visible":bool, "Container Bounds":T1, "Height":u32, "Width":u32, "Is XControl?":bool, "Array Element":refnum<vi>, "HorizScroll":bool, "Index Values":u32[], "Index Visible":bool, "Number of Columns":u32, "NumDims":u32, "Number of Rows":u32, "Selection Size []":u32[], "Selection Start []":u32[], "VertScroll":bool}[], cluster{"ClassID":u32, "ClassName":string, "IsOnBD?":bool, "Owner":cluster{bool, "UID":i32}, "OwningVI":refnum<vi>, "Bounds":T1, "Height":u32, "Width":u32, "Position":T2, "Left":i32, "Top":i32, "Selected":bool, "Bounds Rect":T3, "UID":i32, "Auto-Update":bool, "Desc":string, "Typedef?":enum32{"not a typedef", "typedef", "strict typedef", "class private data"}, "Label":string, "Terminal":i32, "TipStrip":string, "Typedef Path":path, "Typedef VI":refnum<vi>, "Value":variant, "Adapt To Entered Data":bool, "Representation":T7, "DigDisp":refnum<vi>, "Items[]":string[], "Allow Undefined Values?":bool, "Strings And Values[]":T8}[], cluster{"ClassID":u32, "ClassName":string, "IsOnBD?":bool, "Owner":cluster{bool, "UID":i32}, "OwningVI":refnum<vi>, "Bounds":T1, "Height":u32, "Width":u32, "Position":T2, "Left":i32, "Top":i32, "Selected":bool, "Bounds Rect":T3, "UID":i32, "BreakPtStatus":T4, "Desc":string, "Label":string, "Style":string, "Terms[]":i32[], "BadSubVILinkage":bool, "GrowTerms":string[], "SkipSbrtCall":bool, "CloseFPAfterCall":bool, "Open FP On Load":bool, "Show FP On Call":bool, "SuspendOnCall":bool, "TermVis":bool, "VIName":string, "VIPath":path, "VI Ref":refnum<vi>, "ViewAsIcon":bool}[], cluster{"ClassID":u32, "ClassName":string, "IsOnBD?":bool, "Owner":cluster{bool, "UID":i32}, "OwningVI":refnum<vi>, "Bounds":T1, "Height":u32, "Width":u32, "Position":T2, "Left":i32, "Top":i32, "Selected":bool, "Bounds Rect":T3, "UID":i32, "InsideTerms[]":i32[], "Outer Term":i32, "RightReg":i32}[], cluster{"ClassID":u32, "ClassName":string, "IsOnBD?":bool, "Owner":cluster{bool, "UID":i32}, "OwningVI":refnum<vi>, "Bounds":T1, "Height":u32, "Width":u32, "Position":T2, "Left":i32, "Top":i32, "Selected":bool, "Bounds Rect":T3, "UID":i32, "InsideTerms[]":i32[], "Outer Term":i32, "LeftRegs[]":i32[]}[], cluster{"ClassID":u32, "ClassName":string, "IsOnBD?":bool, "Owner":cluster{bool, "UID":i32}, "OwningVI":refnum<vi>, "Bounds":T1, "Height":u32, "Width":u32, "Position":T2, "Left":i32, "Top":i32, "Selected":bool, "Bounds Rect":T3, "UID":i32, "BreakPtStatus":T4, "Desc":string, "Label":string, "Style":string, "Terms[]":i32[], "AutoSize":bool, "Content Rect":T3, "Diagrams":refnum<vi>[], "Fix Contents":bool, "Frame Size":T1, "AutoSharedCloneAllocStrategyEnabled":bool, "PreAllocSharedClones":bool, "SubDiagLbl Vis":bool, "Tunnels[]":i32[], "Diagram":i32, "LpCounter":refnum<vi>, "ShiftRegs[]":i32[], "LpEndRef":refnum<vi>, "StopIfTrue":bool}[], cluster{"ClassID":u32, "ClassName":string, "IsOnBD?":bool, "Owner":cluster{bool, "UID":i32}, "OwningVI":refnum<vi>, "Bounds":T1, "Height":u32, "Width":u32, "Position":T2, "Left":i32, "Top":i32, "Selected":bool, "Bounds Rect":T3, "UID":i32, "BreakPtStatus":T4, "Desc":string, "Label":string, "Style":string, "Terms[]":i32[], "AutoSize":bool, "Content Rect":T3, "Diagrams":refnum<vi>[], "Fix Contents":bool, "Frame Size":T1, "AutoSharedCloneAllocStrategyEnabled":bool, "PreAllocSharedClones":bool, "SubDiagLbl Vis":bool, "Tunnels[]":i32[], "Diagram":i32, "LpCounter":refnum<vi>, "ShiftRegs[]":i32[], "ChunkSizeTunnel":refnum<vi>, "PTunnel":refnum<vi>, "HasConditionalTerm":bool, "DebuggingAllowed":bool, "IsParallelismEnabled":bool, "LpCount":refnum<vi>, "LpEndRef":refnum<vi>, "NumStaticParWorkers":i32, "ParallelSchedule":T9, "StopIfTrue":bool}[], cluster{"ClassID":u32, "ClassName":string, "IsOnBD?":bool, "Owner":cluster{bool, "UID":i32}, "OwningVI":refnum<vi>, "Bounds":T1, "Height":u32, "Width":u32, "Position":T2, "Left":i32, "Top":i32, "Selected":bool, "Bounds Rect":T3, "UID":i32, "AllObjs[]":refnum<vi>[], "BreakPtStatus":T4, "Color":u32, "Decos[]":refnum<vi>[], "FiringOrder":refnum<vi>[], "Nodes[]":refnum<vi>[], "SubDiag Label":refnum<vi>, "SubVIs[]":refnum<vi>[], "Wires[]":refnum<vi>[], "VisBounds":T1}[], cluster{"ClassID":u32, "ClassName":string, "IsOnBD?":bool, "Owner":cluster{bool, "UID":i32}, "OwningVI":refnum<vi>, "Bounds":T1, "Height":u32, "Width":u32, "Position":T2, "Left":i32, "Top":i32, "Selected":bool, "Bounds Rect":T3, "UID":i32, "AllObjs[]":refnum<vi>[], "Controls[]":i32[], "Decos[]":refnum<vi>[], "DeferPanUpdts":bool, "Panes[]":refnum<vi>[], "SelList[]":refnum<vi>[], "Splitters[]":refnum<vi>[]}[], cluster{"ClassID":u32, "ClassName":string, "IsOnBD?":bool, "Owner":cluster{bool, "UID":i32}, "OwningVI":refnum<vi>, "Bounds":T1, "Height":u32, "Width":u32, "Position":T2, "Left":i32, "Top":i32, "Selected":bool, "Bounds Rect":T3, "UID":i32, "InsideTerms[]":i32[], "Outer Term":i32}[]}
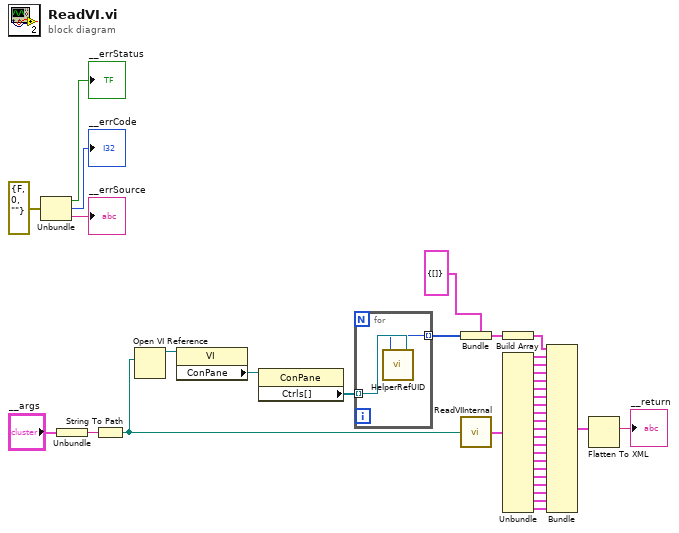
[diagram p0: block diagram]
diagram:
  n1 = Unbundle(errorcluster {"status"=FALSE, "code"=0, "source"=""} ("cluster")) -> ("status"=→"__errStatus":bool, "code"=→"__errCode":i32, "source"=→"__errSource":string)
  n2 = Unbundle("__args") -> ("targetVi"=w32:string)
  n3 = String To Path(string=w32) -> (path=w30:path)
  n4 = Open VI Reference(vi path=w30) -> (vi reference=w10:refnum<vi>)  [unwired: 5 in, 1 out]
  n5 = property class="VI"(reference=w10) -> ("ConPane"=w9:refnum<vi>)  [unwired: 1 in, 2 out]
  n6 = property class="ConPane"(reference=w9) -> ("Ctrls[]"=w8:refnum<vi>[])  [unwired: 1 in, 2 out]
  n7 = for {
    tunnel: w8 -> [w39] mode=indexing
    tunnel: [w38] -> w6 mode=indexing
    n8 = call "HelperRefUID.vi"("Text in"=w39) -> ("UID"=w38:i32)
  }
  n9 = Bundle(cluster=cluster{"Controls[]":i32[]} {"Controls[]"=[]} ("ConnectorPane"), "Controls[]"=w6) -> (w4:cluster{"Controls[]":i32[]})
  n10 = call "ReadVIInternal.vi"("vi path"=w30) -> ("output cluster"=w29:T13)
  n11 = Build Array(w4) -> (w1:cluster{"Controls[]":i32[]}[])
  n12 = Unbundle(w29) -> ("Wire"=w28:T14, w27:T15, w26:T16, w25:T17, w24:T17, w23:T18, w22:T19, w21:T20, w20:T21, w19:T22, w18:T23, w16:T24, w17:T25, w15:T26, w14:T27, w13:T28, w12:T29, w11:T30, w3:T31, w2:T32)
  n13 = Bundle(w1, "Wire"=w28, w27, w26, w25, w24, w23, w22, w21, w20, w19, w18, w16, w17, w15, w14, w13, w12, w11, w3, w2) -> (w7:T33)  [unwired: 1 in]
  n14 = Flatten To XML(anything=w7) -> (xml string=→"__return":string)
